vi "configDB.vi"() -> ()   [LabVIEW 2016]
panel:
  in  "specOffset":dbl
  in  "specMultiplier":dbl
  in  "Init File":path=path "C:/Users/Administrator/Desktop/micro.ini"
  in  "stageOrigin":string
  in  "division":dbl
  in  "stageDivision":string
  in  "focalLength":dbl
  in  "distance":dbl
  in  "floatingDigits":i32
  in  "yRange":dbl
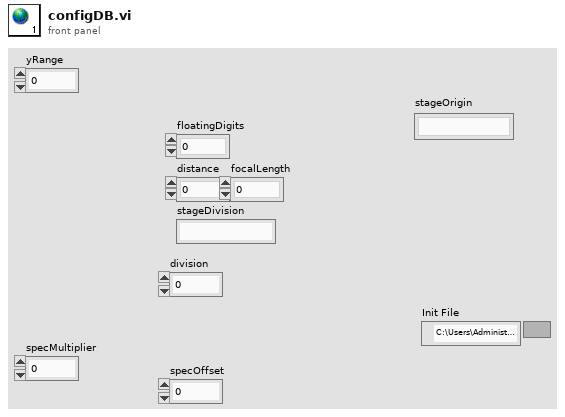
[diagram p1: front panel]
diagram:
